vi "Close.vi"(8 "error in (no error)":errorcluster, 11 "Unit Of Work in":refnum<class "Unit Of Work Session.lvclass">) -> (0 "error out":errorcluster)   [LabVIEW 2020, in "Conditu2.lvlib" / "Unit Of Work Session.lvclass"]
uses:
  Unit Of Work Session.lvclass
  Unit Of Work Session.lvclass/Unit Of Work Session.ctl
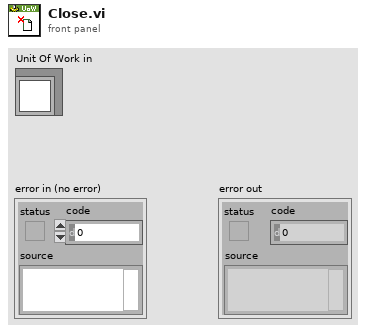
[diagram p1: front panel]
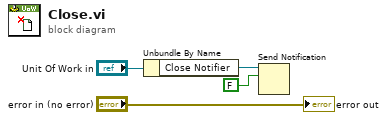
[diagram p0: block diagram]
diagram:
  n1 = Unbundle By Name("Unit Of Work in") -> ("Close Notifier"=w2:refnum<notifier>)
  n2 = Send Notification(notification=FALSE, notifier=w2) -> ()  [unwired: 1 in, 2 out]
  "error out" <- "error in (no error)"
